vi "Hide Python UI.vi"(7 "Server Alias":string, 8 "error in (no error)":errorcluster) -> (0 "error out":errorcluster)   [LabVIEW 2013, in "TS.lvlib"]
doc: "This is a particular message to hide the Python-side GUI, which is not usually necessary for the user to see."
uses:
  TS.lvlib
  LabVIEW Python Connector Message.ctl
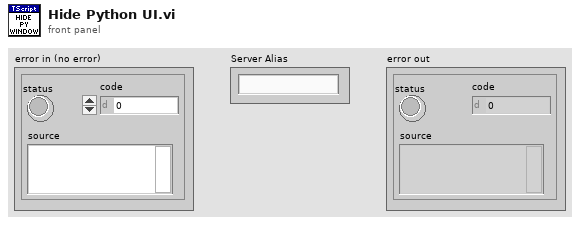
[diagram p1: front panel]
types:
  T1 = typedef "TS.lvlib/LabVIEW Python Connector Message.ctl" = cluster{"Command":string, "Data":string[], "Script ID":i64, "LabVIEW Server ID":string, "Python Message ID":i32}
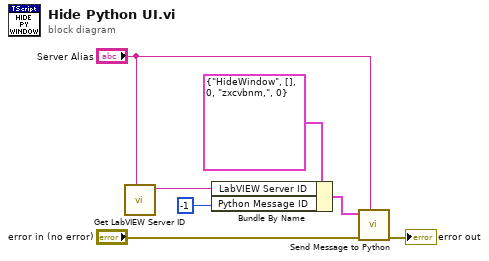
[diagram p0: block diagram]
diagram:
  n1 = call "Get LabVIEW Server ID.vi"("Server Alias"="Server Alias") -> ("LabVIEW Server ID"=w2:string)  [unwired: 9 in, 1 out]
  n2 = Bundle By Name(cluster=T1 {"Command"="HideWindow", "Data"=[], "Script ID"=0, "LabVIEW Server ID"="zxcvbnm,", "Python Message ID"=0} ("Message"), "LabVIEW Server ID"=w2, "Python Message ID"=-1) -> (w4:T1)
  n3 = call "Send Message to Python.vi"("Server Alias"="Server Alias", "error in (no error)"="error in (no error)", "Message"=w4) -> ("error out"=→"error out":errorcluster)  [unwired: 8 in]
